vi "WriteEvtConfigRequest.vi"(8 "error in (no error)":errorcluster, 10 "clEvtConfig":T1={"T0(UTC)"=60.0, "F0"=60.0, "Fs"=0, "FSamp"=0}, 11 "ModuleID":i32=-1) -> (0 "error out":errorcluster)   [LabVIEW 2014, in "WfrmModule.lvlib"]
uses:
  WfrmModule.lvlib
  WfrmPlugins/EventPluginBaseClass/TypeDefs/WfrmConfig.ctl
  clEventType.ctl
  <vilib>/Utility/error.llb/Error Cluster From Error Code.vi
  <vilib>/ErrorRing/Error Ring.xnode
  WfrmPlugins/EventPluginBaseClass/BaseWfrmPlugin.lvclass
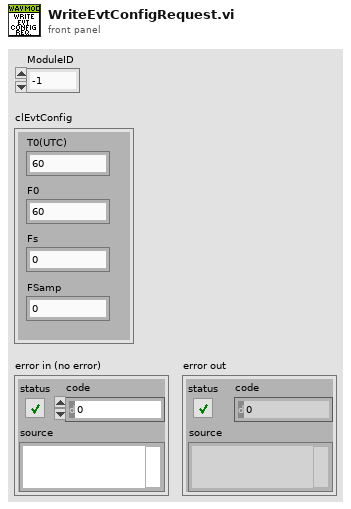
[diagram p1: front panel]
types:
  T1 = typedef "WfrmPlugins.lvlib/BaseWfrmPlugin.lvclass/WfrmConfig.ctl" = cluster{"T0(UTC)":dbl, "F0":dbl, "Fs":i32, "FSamp":u32}
  T2 = typedef "WfrmModule.lvlib/clRequestEvents.ctl" = cluster{"StopRequest":refnum<user-event>, "LoadPluginRequest":refnum<user-event>, "WriteEvtConfig":refnum<user-event>, "ReadEvtConfig":refnum<user-event>, "WriteTimeArray":refnum<user-event>, "ReadTimeArray":refnum<user-event>, "WriteEvtParams":refnum<user-event>, "ReadEvtParams":refnum<user-event>, "GetEvtReportArray":refnum<user-event>, "ReadPathToPlugin":refnum<user-event>, "GetEvtSignal":refnum<user-event>, "SendArbWfrm":refnum<user-event>}
  T3 = typedef "WfrmModule.lvlib/clEventType.ctl" = cluster{"ModuleID":i32, "Data":variant}
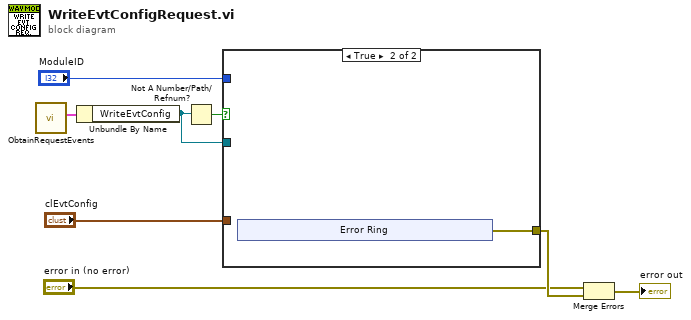
[diagram p0: block diagram]
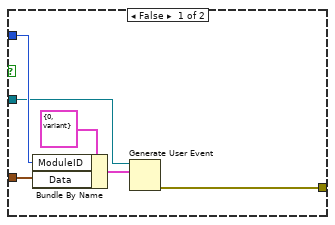
[diagram p2: hidden frame]
diagram:
  n1 = call "ObtainRequestEvents.vi"() -> ("clRequestEvents"=w8:T2)  [unwired: 10 in, 1 out]
  n2 = Unbundle By Name(w8) -> ("WriteEvtConfig"=w6:refnum<user-event>)
  n3 = Not A Number/Path/Refnum?(number/path/refnum=w6) -> (NaN/Path/Refnum?=w7:bool)
  n4 = case shown="True" w7 {
    tunnel: w6 -> [w11 _]
    tunnel: "ModuleID" -> [w13 _]
    tunnel: "clEvtConfig" -> [w12 _]
    tunnel: [w9 w15] -> w2
    frame False {
      n5 = Bundle By Name(cluster=T3 {"ModuleID"=0, "Data"=variant} ("clEventType"), "ModuleID"=w13, "Data"=w12) -> (w10:T3)
      n6 = Generate User Event(user event=w11, event data cluster=w10) -> (error out=w9:errorcluster)  [unwired: 2 in, 1 out]
    }
    frame True {
      n7 = xnode "Error Ring"() -> ("error out"=w15:errorcluster)
    }
  }
  n8 = Merge Errors("error in (no error)", w2) -> (→"error out":errorcluster)
